vi "WaveformDAQ_tb4.vi"() -> ()   [LabVIEW 2018]
uses:
  <vilib>/DAQmx/read.llb/DAQmx Read (Analog Wfm 1Chan NSamp).vi
  <vilib>/DAQmx/create/channels.llb/DAQmx Create Channel (AI-Voltage-Basic).vi
  <vilib>/DAQmx/configure/timing.llb/DAQmx Timing (Sample Clock).vi
  <vilib>/DAQmx/miscellaneous.llb/DAQmx Fill In Error Info.vi
  <instrlib>/Agilent 33XXX Series/Agilent 33XXX Series.lvlib
  <resource>/objmgr/daqmx.rc
panel:
  out "Sample Rate":dbl
  out "Waveform Graph 2":waveform(dbl)(graph)
  in  "Sample Clock Source":tag="OnboardClock"
  out "error out":errorcluster
  out "Actual Sample Rate":dbl=1000.0 format="%0.2f"
  in  "Sample Mode":i32(ring)=10123 items=["Finite Samples"=10178, "Continuous Samples"=10123, "Hardware Timed Single Point"=12522]
  in  "Terminal Configuration":i32(ring)=-1 items=["default"=-1, "RSE"=10083, "NRSE"=10078, "Differential"=10106, "Pseudodifferential"=12529]
  in  "Voltage Max Value":dbl=5.0 caption="Max Value"
  in  "Voltage Min Value":dbl=-5.0 caption="Min Value"
  in  "Voltage Physical Channels":tag="Dev1/ai0" caption="Physical Channels"
  in  "stop":bool
  out "Waveform Graph":waveform(dbl)(graph)
  in  "Amplitude (1 Vpp)":dbl=1.0
  in  "DC Offset (0.00 V)":dbl
  in  "Waveform Function (1: Sine)":u16(ring)=1 items=["DC", "Sine", "Square", "Triangle", "Ramp", "Pulse", "Noise", "Sinc", "Negative Ramp", "Exponential Rise", "Exponential Fall", "Cardiac"]
  in  "Frequency (1000 Hz)":dbl=1000.0
  in  "Sample rate":enum16{"1KHz", "10KHz", "100KHz", "1MHz"}(ring)
  in  "Time":dbl
  out "N Samples":dbl
  in  "Serial Configuration":T1={"Baud Rate"=9600, "Parity"=0, "Data Bits"=8, "Flow Control"=4} {"Flow Control" items=["None", "XON/XOFF", "RTS/CTS", "XON/XOFF & RTS/CTS", "DTR/DSR", "XON/XOFF & DTR/DSR"]; "Data Bits" items=["7"=7, "8"=8]; "Parity" items=["None", "Odd", "Even", "Mark", "Space"]; "Baud Rate" items=["300"=300, "600"=600, "1200"=1200, "2400"=2400, "4800"=4800, "9600"=9600, "19200"=19200]}
  in  "VISA resource name":refnum<visa-resource-name>
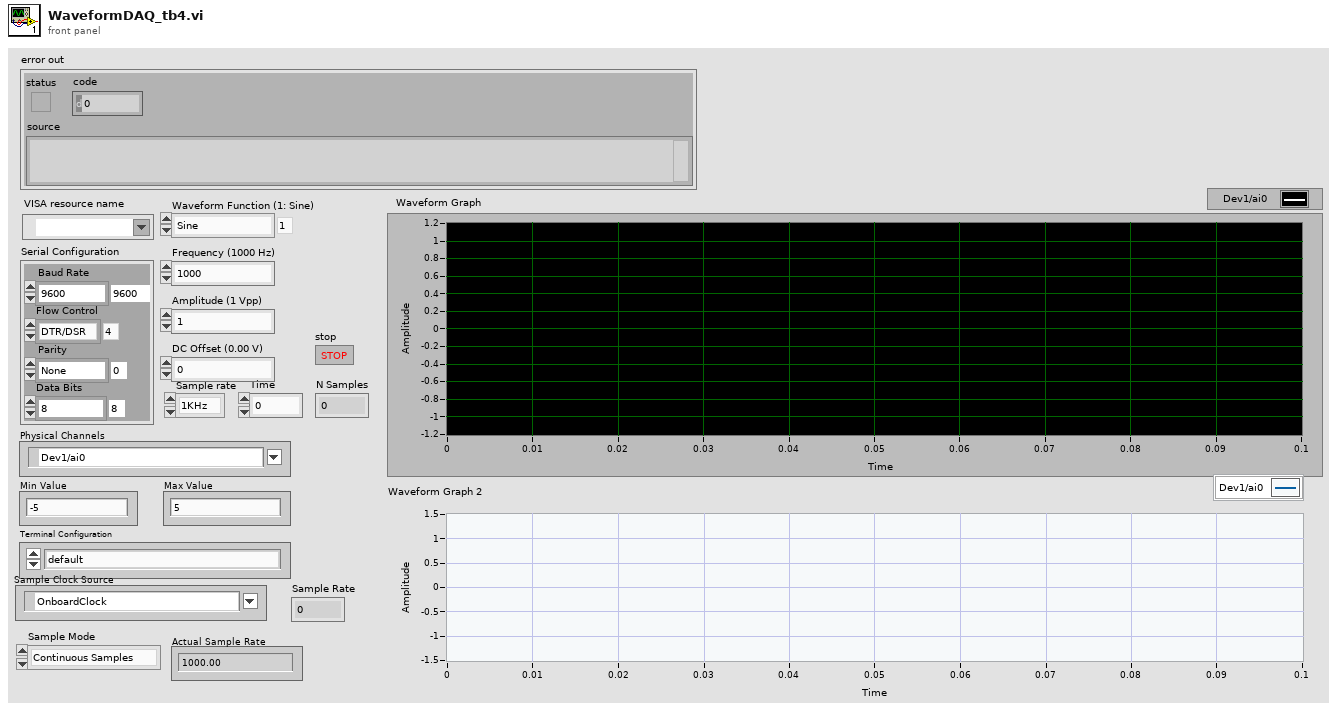
[diagram p1: front panel]
types:
  T1 = cluster{"Baud Rate":u32, "Parity":u16, "Data Bits":u16, "Flow Control":u16}
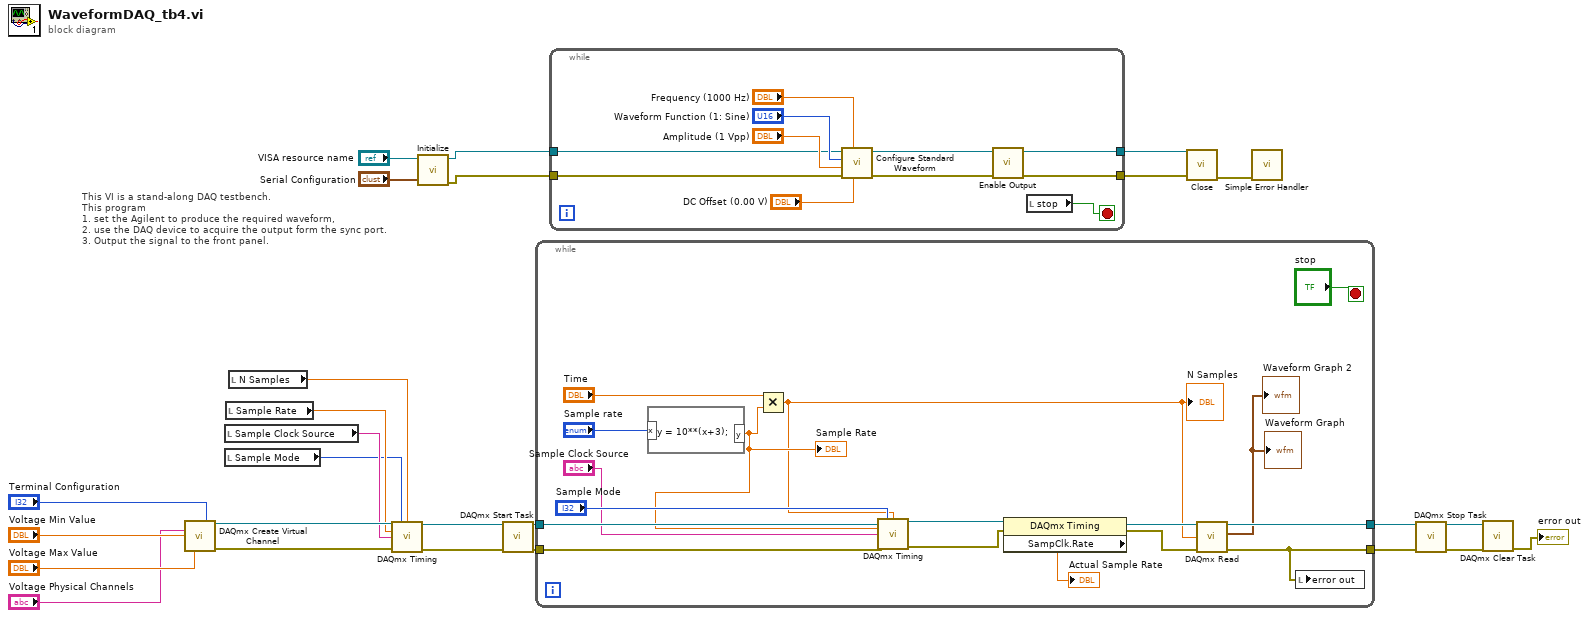
[diagram p0: block diagram]
diagram:
  # "This VI is a stand-along DAQ testbench.  \nThis program \n1. set the Agilent to produce the required waveform,\n2. use the DAQ device to acquire the output form the sync port. \n3. Output the signal to the front panel."
  n1 = call-poly <vilib>:"DAQmx Create Virtual Channel.vi"("maximum value"="Voltage Max Value", "minimum value"="Voltage Min Value", "input terminal configuration"="Terminal Configuration", "physical channels"="Voltage Physical Channels") -> ("task out"=w10:refnum<k21>, "error out"=w9:errorcluster)  [unwired: 10 in]
  n2 = local read "Sample Clock Source"() -> (w8:tag)
  n3 = local read "Sample Mode"() -> (w6:i32)
  n4 = local read "Sample Rate"() -> (w7:dbl)
  n5 = local read "N Samples"() -> (w5:dbl)
  n6 = call-poly <vilib>:"DAQmx Timing.vi"("task/channels in"=w10, "sample mode"=w6, "samples per channel"=w5, "rate"=w7, "source"=w8, "error in"=w9) -> ("task out"=w11:refnum<k21>, "error out"=w12:errorcluster)  [unwired: 8 in]
  n7 = call <instrlib>:"Initialize.vi"("Serial Configuration"="Serial Configuration", "VISA resource name"="VISA resource name") -> ("error out"=w3:errorcluster, "VISA resource name out"=w4:refnum<visa-resource-name>)  [unwired: 8 in]
  n8 = call <vilib>:"DAQmx Start Task.vi"("task/channels in"=w11, "error in"=w12) -> ("task out"=w19:refnum<k21>, "error out"=w18:errorcluster)  [unwired: 12 in]
  n9 = while {
    tunnel: w19 -> [w38]
    tunnel: w18 -> [w37]
    tunnel: [w42] -> w17
    tunnel: [w28] -> w16
    stop <- "stop" stop-if-true
    n10 = formula code="y = 10**(x+3);"("x"="Sample rate") -> ("y"=w35:dbl)
    "Sample Rate" <- w35
    n11 = Multiply(x="Time", y=w35) -> (x*y=w27:dbl)
    "N Samples" <- w27
    n12 = call-poly <vilib>:"DAQmx Timing.vi"("task/channels in"=w38, "sample mode"="Sample Mode", "samples per channel"=w27, "rate"=w35, "source"="Sample Clock Source", "error in"=w37) -> ("task out"=w33:refnum<k21>, "error out"=w29:errorcluster)  [unwired: 8 in]
    n13 = property class="DAQmx Timing"(reference=w33, error in=w29) -> (reference out=w32:refnum<k21>, error out=w31:errorcluster, "SampClk.Rate"=→"Actual Sample Rate":dbl)
    n14 = call-poly <vilib>:"DAQmx Read.vi"("task/channels in"=w32, "number of samples per channel"=w27, "error in"=w31) -> ("task out"=w42:refnum<k21>, "data"=→"Waveform Graph" →"Waveform Graph 2":waveform(dbl), "error out"=w28:errorcluster)  [unwired: 10 in]
    n15 = local write "error out"(w28) -> ()
  }
  n16 = while {
    tunnel: w4 -> [w47]
    tunnel: w3 -> [w46]
    tunnel: [w45] -> w2
    tunnel: [w44] -> w1
    stop <- w48 stop-if-true
    n17 = call <instrlib>:"Configure Standard Waveform.vi"("DC Offset (0.00 V)"="DC Offset (0.00 V)", "Frequency (1000 Hz)"="Frequency (1000 Hz)", "error in (no error)"=w46, "Amplitude (1)"="Amplitude (1 Vpp)", "Waveform Function (1: Sine)"="Waveform Function (1: Sine)", "VISA resource name"=w47) -> ("error out"=w50:errorcluster, "VISA resource name out"=w51:refnum<visa-resource-name>)  [unwired: 4 in]
    n18 = call <instrlib>:"Enable Output.vi"("error in (no error)"=w50, "VISA resource name"=w51) -> ("error out"=w44:errorcluster, "VISA resource name out"=w45:refnum<visa-resource-name>)  [unwired: 8 in]
    n19 = local read "stop"() -> (w48:bool)
  }
  n20 = call <instrlib>:"Close.vi"("error in (no error)"=w1, "VISA resource name"=w2) -> ("error out"=w25:errorcluster)  [unwired: 9 in]
  n21 = call <vilib>:"Simple Error Handler.vi"("error in (no error)"=w25) -> ()  [unwired: 4 in, 5 out]
  n22 = call <vilib>:"DAQmx Stop Task.vi"("task/channels in"=w17, "error in"=w16) -> ("task out"=w15:refnum<k21>, "error out"=w14:errorcluster)  [unwired: 12 in]
  n23 = call <vilib>:"DAQmx Clear Task.vi"("task in"=w15, "error in"=w14) -> ("error out"=→"error out":errorcluster)  [unwired: 13 in]
